vi "ReadWfmFromDAQ.vi"(8 "error in":errorcluster, 10 "clock settings":T1={"sample mode"=10178, "samples per channel"=1000, "rate"=1000.0} {"sample mode" items=["Finite Samples"=10178, "Continuous Samples"=10123, "Hardware Timed Single Point"=12522]}, 11 "channel settings":T2={"max value"=5.0, "min value"=-5.0, "physical channels"="Dev1/ai2", "input terminal configuration"=-1, "units"=10348} {"input terminal configuration" items=["Default"=-1, "RSE"=10083, "NRSE"=10078, "Differential"=10106, "Pseudodifferential"=12529]; "units" items=["Volts"=10348, "From Custom Scale"=10065]}) -> (0 "error out":errorcluster, 3 "data":waveform(dbl)(graph))   [LabVIEW 2025]
uses:
  <vilib>/DAQmx/create/channels.llb/DAQmx Create Channel (AI-Voltage-Basic).vi
  <vilib>/DAQmx/configure/timing.llb/DAQmx Timing (Sample Clock).vi
  <vilib>/DAQmx/miscellaneous.llb/DAQmx Fill In Error Info.vi
  <vilib>/DAQmx/read.llb/DAQmx Read (Analog Wfm 1Chan NSamp).vi
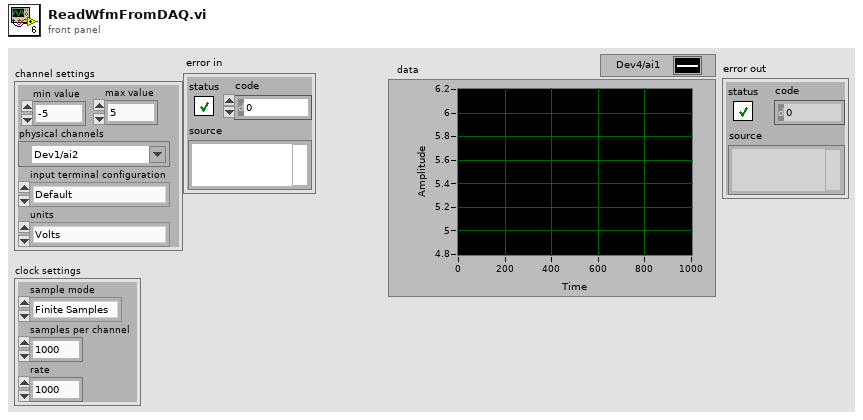
[diagram p1: front panel]
types:
  T1 = cluster{"sample mode":i32, "samples per channel":i32, "rate":dbl}
  T2 = cluster{"max value":dbl, "min value":dbl, "physical channels":tag, "input terminal configuration":i32, "units":i32}
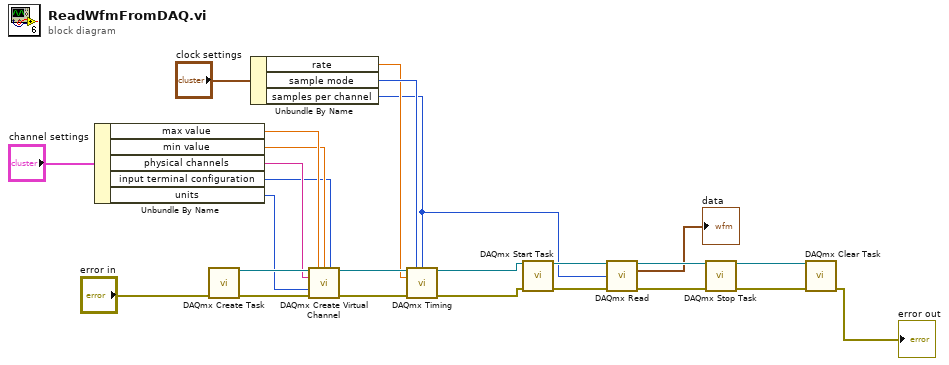
[diagram p0: block diagram]
diagram:
  n1 = Unbundle By Name("channel settings") -> ("max value"=w17:dbl, "min value"=w16:dbl, "physical channels"=w18:tag, "input terminal configuration"=w15:i32, "units"=w14:i32)
  n2 = call <vilib>:"DAQmx Create Task.vi"("error in"="error in") -> ("task out"=w24:refnum<k21>, "error out"=w23:errorcluster)  [unwired: 13 in]
  n3 = Unbundle By Name("clock settings") -> ("rate"=w13:dbl, "sample mode"=w20:i32, "samples per channel"=w2:i32)
  n4 = call-poly <vilib>:"DAQmx Create Virtual Channel.vi"("task in"=w24, "maximum value"=w17, "minimum value"=w16, "input terminal configuration"=w15, "physical channels"=w18, "units"=w14, "error in"=w23) -> ("task out"=w25:refnum<k21>, "error out"=w22:errorcluster)  [unwired: 7 in]
  n5 = call-poly <vilib>:"DAQmx Timing.vi"("task/channels in"=w25, "sample mode"=w20, "samples per channel"=w2, "rate"=w13, "error in"=w22) -> ("task out"=w6:refnum<k21>, "error out"=w5:errorcluster)  [unwired: 9 in]
  n6 = call <vilib>:"DAQmx Start Task.vi"("task/channels in"=w6, "error in"=w5) -> ("task out"=w8:refnum<k21>, "error out"=w7:errorcluster)  [unwired: 12 in]
  n7 = call-poly <vilib>:"DAQmx Read.vi"("task/channels in"=w8, "number of samples per channel"=w2, "error in"=w7) -> ("task out"=w10:refnum<k21>, "data"=→"data":waveform(dbl), "error out"=w9:errorcluster)  [unwired: 10 in]
  n8 = call <vilib>:"DAQmx Stop Task.vi"("task/channels in"=w10, "error in"=w9) -> ("task out"=w12:refnum<k21>, "error out"=w11:errorcluster)  [unwired: 12 in]
  n9 = call <vilib>:"DAQmx Clear Task.vi"("task in"=w12, "error in"=w11) -> ("error out"=→"error out":errorcluster)  [unwired: 13 in]
